vi "ExecuteRun.vi"(8 "error in (no error)":errorcluster, 10 "Drona Tests PPL":path, 11 "EXE Path":path) -> (0 "error out":errorcluster)   [LabVIEW 2016, in "Drona.lvlib"]
doc: "Launches EXE and initiates the Run VI present in the given Drona Tests packed project library path"
uses:
  Drona.lvlib
  Get/GetVI/GetVIByPath.vi
  Stimulus/VI/RunVI.vi
  Get/GetVI/GetVI.lvlib
  Stimulus/VI/VI.lvlib
  <vilib>/SLL Toolkit/SLL File IO/SLL File IO.lvlib
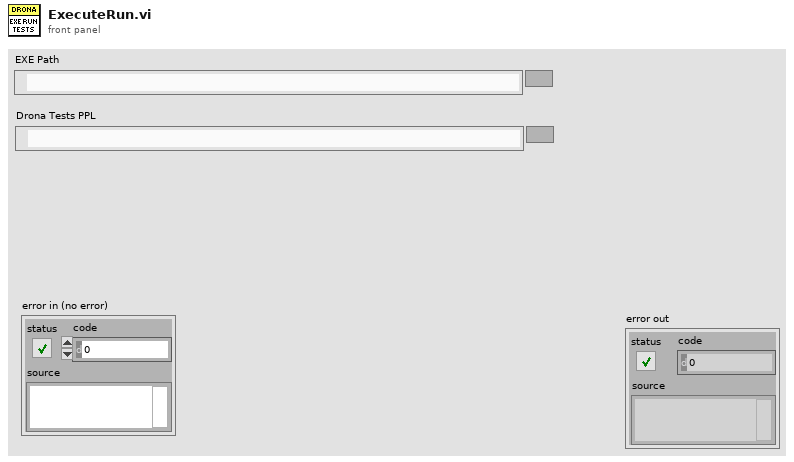
[diagram p1: front panel]
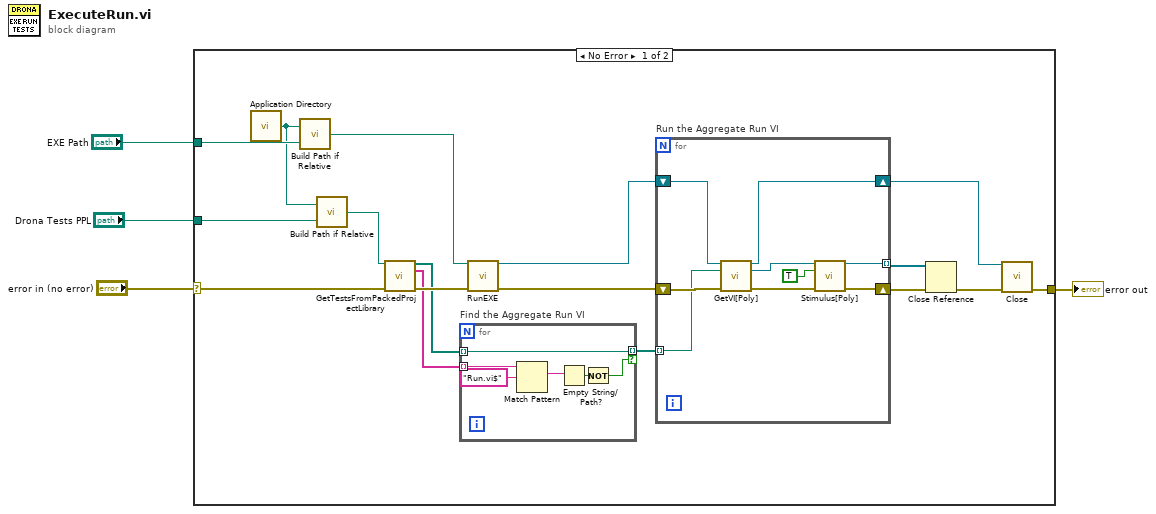
[diagram p0: block diagram]
diagram:
  n1 = case shown="No Error" "error in (no error)" {
    selector: "error in (no error)" -> [w16 w37]
    tunnel: "Drona Tests PPL" -> [w6 _]
    tunnel: "EXE Path" -> [w9 _]
    tunnel: [w17 w37] -> w2
    frame No Error {
      n2 = call <vilib>:"Application Directory.vi"() -> ("Application Directory"=w5:path)
      n3 = call <vilib>:"Build Path if Relative.vi"("Relative or Absolute Path"=w9, "Base Path"=w5) -> ("Path Out"=w8:path)
      n4 = call <vilib>:"Build Path if Relative.vi"("Relative or Absolute Path"=w6, "Base Path"=w5) -> ("Path Out"=w7:path)
      n5 = call "GetTestsFromPackedProjectLibrary.vi"("Packed Project Library Path"=w7, "error in (no error)"=w16) -> ("Tests"=w12:path[], "Qualified Names"=w11:string[], "error out"=w18:errorcluster)  [unwired: 11 in]
      n6 = for "Find the Aggregate Run VI" {
        tunnel: w12 -> [w24] mode=indexing
        tunnel: w11 -> [w27] mode=indexing
        tunnel: [w24] -> w10 mode=indexing if=w22
        n7 = Match Pattern(string=w27, regular expression="Run.vi$") -> (match substring=w25:string)  [unwired: 1 in, 3 out]
        n8 = Empty String/Path?(string/path=w25) -> (empty?=w23:bool)
        n9 = Not(x=w23) -> (.not. x?=w22:bool)
      }
      n10 = call "RunEXE.vi"("EXE Path"=w8, "error in (no error)"=w18) -> ("Application Ref"=w15:refnum<vi>, "error out"=w19:errorcluster)  [unwired: 12 in]
      n11 = for "Run the Aggregate Run VI" {
        shift-right: [w33] -> w21
        shift-left: w19 -> [w32]
        tunnel: w10 -> [w31] mode=indexing
        shift-right: [w30] -> w20
        shift-left: w15 -> [w36]
        tunnel: [w28] -> w13 mode=indexing
        n12 = call-poly "GetVI[Poly].vi"("Application Ref in"=w36, "VI Path"=w31, "error in (no error)"=w32) -> ("Application Ref out"=w30:refnum<vi>, "VI Reference"=w35:refnum<vi>, "error out"=w34:errorcluster)  [unwired: 10 in]
        n13 = call-poly "Stimulus[Poly].vi"("VI Reference In"=w35, "Wait Until Done (F)"=TRUE, "error in"=w34) -> ("VI Reference Out"=w28:refnum<vi>, "error out"=w33:errorcluster)  [unwired: 11 in]
      }
      n14 = Close Reference(reference=w13, error in (no error)=w21) -> (error out=w14:errorcluster)
      n15 = call "Close.vi"("Application Ref"=w20, "error in"=w14) -> ("error out"=w17:errorcluster)  [unwired: 13 in]
    }
    frame Error {
    }
  }
  "error out" <- w2
